vi "Ident_temp.vi"() -> ()   [LabVIEW 2020]
uses:
  <vilib>/addons/control/pid/NI_PID_pid.lvlib
  <vilib>/addons/control/pid/pid.llb/PID Advanced (DBL).vi
panel:
  out "Courbes":cluster{dbl, "output":dbl, "Consigne":dbl}(graph)
  out "Cluster sortie":cluster{dbl, "Ser point":dbl}
  in  "PID gains":T1={"proportional gain (Kc)"=1.0, "integral time (Ti, min)"=0.01, "derivative time (Td, min)"=0.0} {"derivative time (Td, min)" format="%.3f"; "integral time (Ti, min)" format="%.3f"; "proportional gain (Kc)" format="%.3f"}
  in  "Bouton Stop":bool
  in  "Consigne":dbl(knob) scale=0.0..80.0
  out "Température":dbl(slide) scale=0.0..80.0
  # "Entrées"
  # "Sorties"
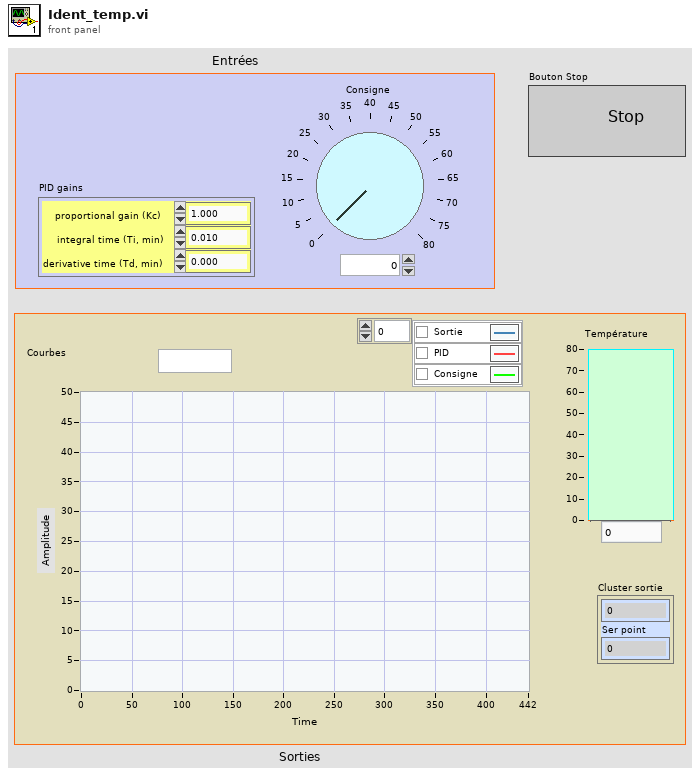
[diagram p1: front panel]
types:
  T1 = cluster{"proportional gain (Kc)":dbl, "integral time (Ti, min)":dbl, "derivative time (Td, min)":dbl}
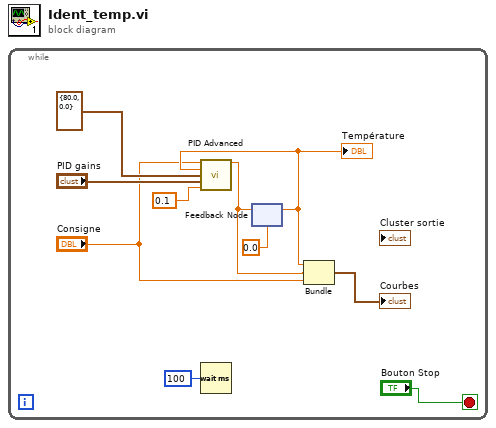
[diagram p0: block diagram]
diagram:
  n1 = while {
    stop <- "Bouton Stop" stop-if-true
    n2 = Wait (ms)(milliseconds to wait=u32 100) -> ()  [unwired: 1 out]
    n3 = feedback #1(0.0) -> (w6:dbl)
    "Température" <- w6
    n4 = call-poly <vilib>:"PID Advanced.vi"("setpoint"="Consigne", "process variable"=w6, "setpoint range"=cluster{"setpoint high":dbl, "setpoint low":dbl} {"setpoint high"=80.0, "setpoint low"=0.0}, "PID gains"="PID gains", "dt (s)"=0.1) -> ("output"=w1:dbl)  [unwired: 9 in, 1 out]
    n5 = feedback-in #1(w1) -> ()
    n6 = Bundle(w6, "output"=w1, "Consigne"="Consigne") -> (→"Courbes":cluster{dbl, "output":dbl, "Consigne":dbl})  [unwired: 1 in]
  }
